vi "Save.vi"(8 "Error In":errorcluster, 9 "Text":string, 11 "reference in":refnum<class "JSONTextViewer.lvclass">) -> (0 "Error Out":errorcluster, 3 "reference in":refnum<class "JSONTextViewer.lvclass">)   [LabVIEW 2021, in "JSONTextViewer.lvlib" / "JSONTextViewer.lvclass"]
uses:
  JSONTextViewer.lvclass
  .Externals/Interface_TAF_IApplicationConfiguration/IApplicationConfiguration/IApplicationConfiguration.lvclass
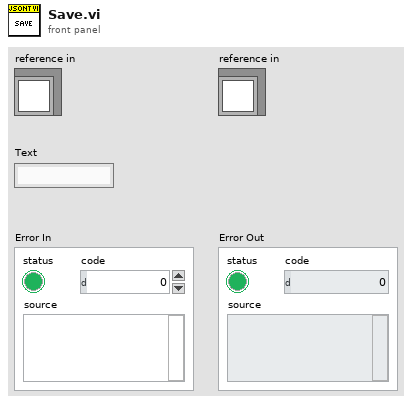
[diagram p1: front panel]
types:
  T1 = typedef "JSONTextViewer.lvlib/JSONTextViewer.lvclass/ObjectAttributes.ctl" = cluster{"Interfaces":cluster{"ApplicationConfiguration":refnum<class "IApplicationConfiguration.lvclass">}, "Locals":cluster{"MainGUIActive":refnum<queue>, "JSONText":string, "ID":string}, "Persistent":cluster{"Dummy":bool}}
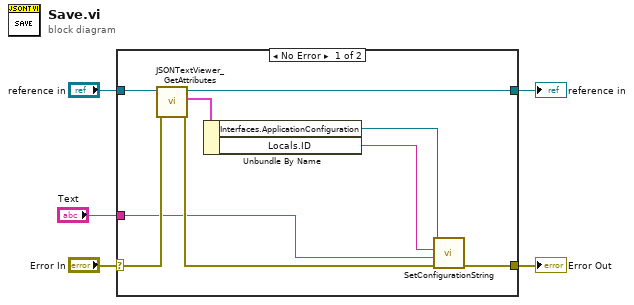
[diagram p0: block diagram]
diagram:
  n1 = case shown="No Error" "Error In" {
    selector: "Error In" -> [w14 w16]
    tunnel: [w9 w16] -> w4
    tunnel: [w10 w15] -> w2
    tunnel: "reference in" -> [w11 w15]
    tunnel: "Text" -> [w6 _]
    frame No Error {
      n2 = call "JSONTextViewer_GetAttributes.vi"("error in (no error)"=w14, "reference in"=w11) -> ("error out"=w12:errorcluster, "Data"=w13:T1, "reference out"=w10:refnum<class "JSONTextViewer.lvclass">)  [unwired: 6 in, 1 out]
      n3 = Unbundle By Name(w13) -> ("Interfaces.ApplicationConfiguration"=w8:refnum<class "IApplicationConfiguration.lvclass">, "Locals.ID"=w7:string)
      n4 = call-dynamic "SetConfigurationString.vi"("Error In"=w12, "String"=w6, "Identification"=w7, "reference in"=w8) -> ("Error Out"=w9:errorcluster)  [unwired: 6 in, 1 out]
    }
    frame Error {
    }
  }
  "Error Out" <- w4
  "reference in" <- w2
